vi "Logger.PGSQL.Connect.vi"(8 "error in (no error)":errorcluster, 11 "Logger.PGSQL in":refnum<class "Logger.PGSQL.lvclass">) -> (0 "error out":errorcluster, 3 "Logger.PGSQL out":refnum<class "Logger.PGSQL.lvclass">)   [LabVIEW 2019, in "Logger.PGSQL.lvlib" / "Logger.PGSQL.lvclass"]
uses:
  Logger.PGSQL.lvclass
  Logger.PGSQL.lvclass/Logger.PGSQL.ctl
  <userlib>/LevyLab/LV-Data/LV-Data.PG/LV-Data.PGSQL.lvclass
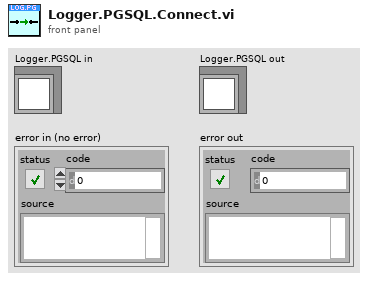
[diagram p1: front panel]
types:
  T1 = enum16{"unconfigured", "disconnected", "connected"}
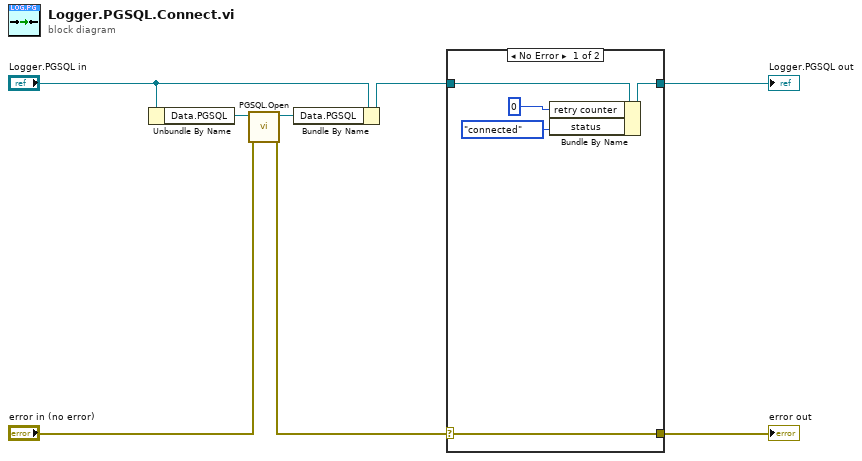
[diagram p0: block diagram]
diagram:
  n1 = Unbundle By Name("Logger.PGSQL in") -> ("Data.PGSQL"=w6:refnum<class "LV-Data.PGSQL.lvclass">)
  n2 = call <userlib>:"PGSQL.Open.vi"("error in (no error)"="error in (no error)", "Data.PG in"=w6) -> ("error out"=w1:errorcluster, "Data.PG out"=w8:refnum<class "LV-Data.PGSQL.lvclass">)  [unwired: 8 in]
  n3 = Bundle By Name(cluster="Logger.PGSQL in", "Data.PGSQL"=w8) -> (w4:refnum<class "Logger.PGSQL.lvclass">)
  n4 = case shown="No Error" w1 {
    selector: w1 -> [w11 w14]
    tunnel: w4 -> [w13 w15]
    tunnel: [w12 w15] -> w3
    tunnel: [w11 w14] -> w2
    frame No Error {
      n5 = Bundle By Name(cluster=w13, "retry counter"=0 ("DB Retries"), "status"=T1."connected") -> (w12:refnum<class "Logger.PGSQL.lvclass">)
    }
    frame Error {
    }
  }
  "Logger.PGSQL out" <- w3
  "error out" <- w2
